vi "Read Key.vi"   [LabVIEW 2020, in "Generic Config Handling.lvlib"]
doc: "This vi reads a variant to a config file.\n\nIt only accepts very basic datatypes. \n\nIt will accept 1D and 2D arrays.\n\nIf key name is not wired, then it will use the name of the section element.\n\nSection Element in provides the type information and the default value."
uses:
  Generic Config Handling.lvlib
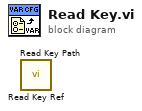
[diagram p0: block diagram]
diagram:
  n1 = call "Read Key Ref.vi"() -> ()  [unwired: 7 in, 5 out]
  n2 = call "Read Key Path.vi"() -> ()  [unwired: 7 in, 5 out]
